vi "Eth Status Read Start_com.vi"(7 "Status Reference":T1, 8 "error in (no error)":errorcluster) -> (0 "error out":errorcluster, 1 "Start":bool, 2 "Stop":bool)   [LabVIEW 2019, in "Eth Status.lvlib"]
uses:
  Eth Status.lvlib
  Ctl/ICPCON Status.ctl
  MB_TCP2/MB_TCP_State.ctl
  MB_TCP2/MB_TCP.lvclass
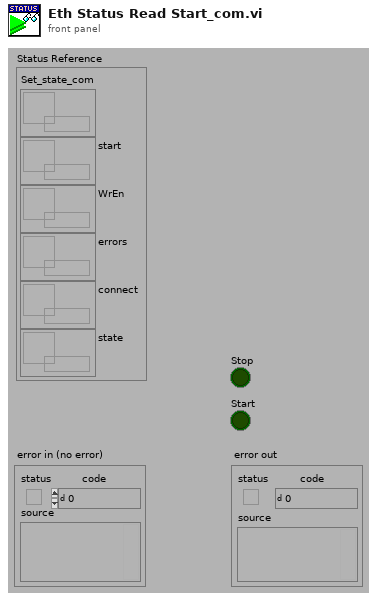
[diagram p1: front panel]
types:
  T1 = typedef "Eth Status.lvlib/ICPCON Status.ctl" = cluster{"Set_state_com":refnum<data-value>, "start":refnum<data-value>, "WrEn":refnum<data-value>, "errors":refnum<data-value>, "connect":refnum<data-value>, "state":refnum<data-value>}
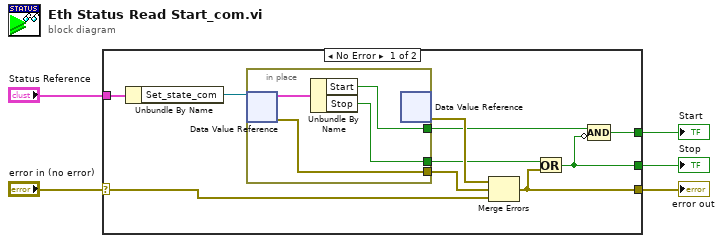
[diagram p0: block diagram]
diagram:
  n1 = case shown="No Error" "error in (no error)" {
    selector: "error in (no error)" -> [w6 w20]
    tunnel: [w7 w20] -> w5
    tunnel: [w9 _] -> w3
    tunnel: "Status Reference" -> [w15 _]
    tunnel: [w8 _] -> w2
    frame No Error {
      n2 = Unbundle By Name(w15) -> ("Set_state_com"=w14:refnum<data-value>)
      n3 = in-place {
        in-place-border: [w19] -> w12
        in-place-border: [w17] -> w11
        in-place-border: [w16] -> w10
        n4 = in-place-dvr #1(w14) -> (w18:cluster{"Start":bool, "WrEn":bool, "Stop":bool}, w19:errorcluster)
        n5 = Unbundle By Name(w18) -> ("Start"=w17:bool, "Stop"=w16:bool)
        n6 = in-place-dvr #1() -> (w13:errorcluster)  [unwired: 1 in, 1 out]
      }
      n7 = Merge Errors(w13, w12, w6) -> (w7:errorcluster)
      n8 = Or(x=w10, y=w7) -> (x .or. y?=w8:bool)
      n9 = Compound Arithmetic op=AND(w11, invert w8) -> (w9:bool)
    }
    frame Error {
    }
  }
  "error out" <- w5
  "Start" <- w3
  "Stop" <- w2
